vi "Convert Unit (DBL Array).vi"(4 "Quantity":T1, 5 "error in (no error)":errorcluster, 6 "Target Unit":T2, 7 "Base Unit":T2, 8 "Data":dbl[](array[numeric])) -> (0 "error out":errorcluster, 3 "Converted Data":dbl[](array[numeric]))   [LabVIEW 2023, in "NI_HFNetworkAnalysis.lvlib"]
doc: "Convert an array of double values for a specified quantity from a base unit to a new unit."
uses:
  NI_HFNetworkAnalysis.lvlib
  Controls/Unit.ctl
  Controls/Quantity.ctl
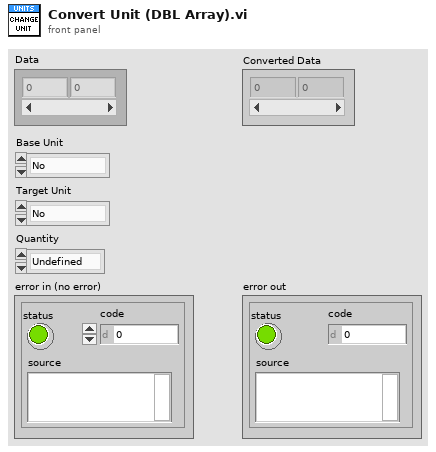
[diagram p1: front panel]
types:
  T1 = typedef "NI_HFNetworkAnalysis.lvlib/Quantity.ctl" = enum16{"Undefined", "V", "I", "A", "B", "P", "Z", "PowerRatio", "Gamma", "Index"}
  T2 = typedef "NI_HFNetworkAnalysis.lvlib/Unit.ctl" = enum16{"No", "s", "Hz", "V", "A", "Ohm", "W", "dB", "dBV", "dBA", "dBm", "percent", "rad", "deg"}
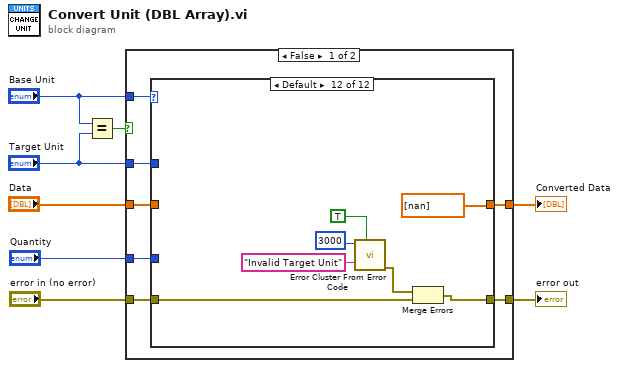
[diagram p0: block diagram]
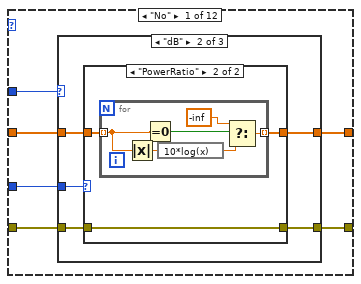
[diagram p2: hidden frame]
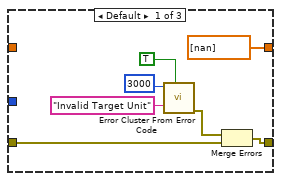
[diagram p3: hidden frame]
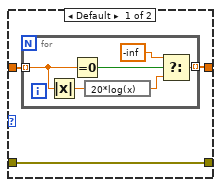
[diagram p4: hidden frame]
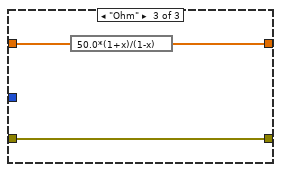
[diagram p5: hidden frame]
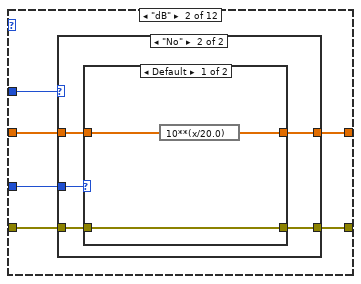
[diagram p6: hidden frame]
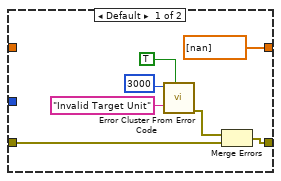
[diagram p7: hidden frame]
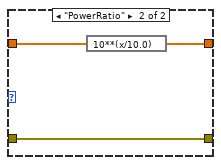
[diagram p8: hidden frame]
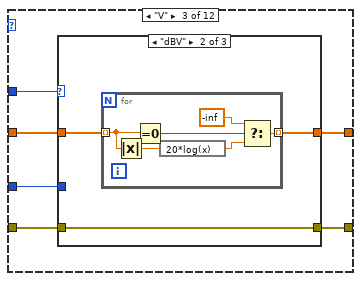
[diagram p9: hidden frame]
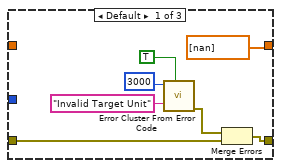
[diagram p10: hidden frame]
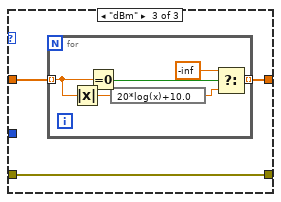
[diagram p11: hidden frame]
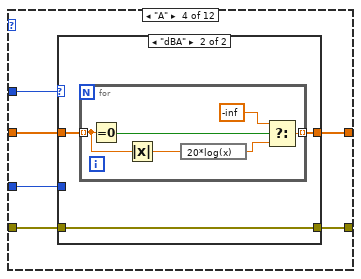
[diagram p12: hidden frame]
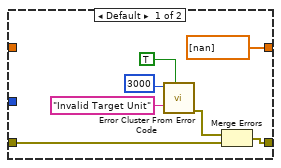
[diagram p13: hidden frame]
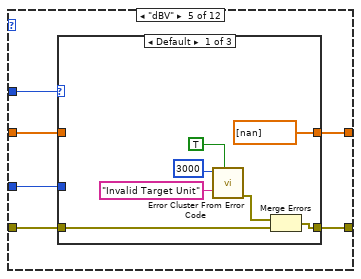
[diagram p14: hidden frame]
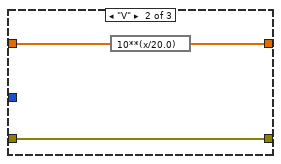
[diagram p15: hidden frame]
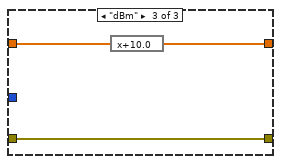
[diagram p16: hidden frame]
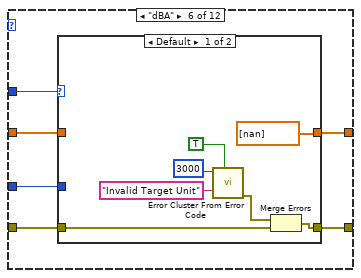
[diagram p17: hidden frame]
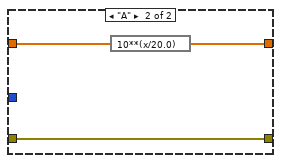
[diagram p18: hidden frame]
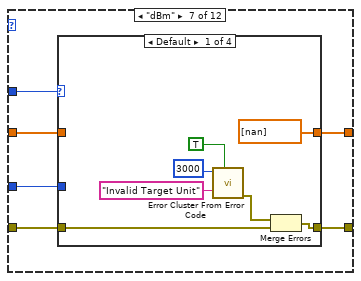
[diagram p19: hidden frame]
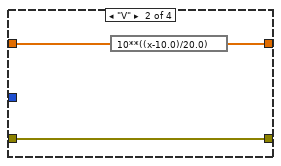
[diagram p20: hidden frame]
diagram:
  n1 = Equal?(x="Base Unit", y="Target Unit") -> (x = y?=w8:bool)
  n2 = case shown="False" w8 {
    tunnel: "Base Unit" -> [w15 _]
    tunnel: [w10 w267] -> w5
    tunnel: "Data" -> [w11 w267]
    tunnel: "Quantity" -> [w14 _]
    tunnel: "error in (no error)" -> [w13 w266]
    tunnel: [w12 w266] -> w2
    tunnel: "Target Unit" -> [w9 _]
    frame False {
      n3 = case shown="Default" w15 {
        tunnel: w14 -> [w21 w60 w84 w115 w137 w156 w172 w194 w215 w231 w247 _]
        tunnel: w13 -> [w20 w59 w83 w114 w136 w155 w171 w193 w214 w230 w246 w265]
        tunnel: [w19 w58 w82 w113 w135 w154 w170 w192 w213 w229 w245 w264] -> w12
        tunnel: w11 -> [w18 w57 w81 w112 w134 w153 w169 w191 w212 w228 w244 _]
        tunnel: [w17 w56 w80 w111 w133 w152 w168 w190 w211 w227 w243 dbl[] [nan] ("Data")] -> w10
        tunnel: w9 -> [w16 w55 w79 w110 w132 w151 w167 w189 w210 w226 w242 _]
        frame "No" {
          n4 = case shown="\"dB\"" w16 {
            tunnel: w21 -> [_ w33 _]
            tunnel: w20 -> [w27 w32 w52]
            tunnel: [w28 w31 w52] -> w19
            tunnel: w18 -> [_ w30 w54]
            tunnel: [dbl[] [nan] ("Data") w29 w53] -> w17
            frame Default {
              n5 = call <vilib>:"Error Cluster From Error Code.vi"("show call chain? (False)"=TRUE, "error message (\"\")"="Invalid Target Unit" ("error message (\"\")"), "error code (0)"=3000) -> ("error out"=w26:errorcluster)  [unwired: 6 in]
              n6 = Merge Errors(w26, w27) -> (w28:errorcluster)
            }
            frame "dB" {
              n7 = case shown="\"PowerRatio\"" w33 {
                tunnel: [w36 w45] -> w31
                tunnel: w32 -> [w36 w45]
                tunnel: w30 -> [w34 w44]
                tunnel: [w35 w43] -> w29
                frame Default {
                  n8 = for {
                    tunnel: [w41] -> w35 mode=indexing
                    tunnel: w34 -> [w38] mode=indexing
                    n9 = Absolute Value(x=w38) -> (abs(x)=w42:dbl)
                    n10 = Equal To 0?(x=w38) -> (x = 0?=w39:bool)
                    n11 = expression code="20*log(x)"(w42) -> (w40:dbl)
                    n12 = Select(t=-inf, s=w39, f=w40) -> (s? t:f=w41:dbl)
                  }
                }
                frame "PowerRatio" {
                  n13 = for {
                    tunnel: w44 -> [w50] mode=indexing
                    tunnel: [w49] -> w43 mode=indexing
                    n14 = Absolute Value(x=w50) -> (abs(x)=w51:dbl)
                    n15 = Equal To 0?(x=w50) -> (x = 0?=w47:bool)
                    n16 = expression code="10*log(x)"(w51) -> (w48:dbl)
                    n17 = Select(t=-inf, s=w47, f=w48) -> (s? t:f=w49:dbl)
                  }
                }
              }
            }
            frame "Ohm" {
              n18 = expression code="50.0*(1+x)/(1-x)"(w54) -> (w53:dbl[])
            }
          }
        }
        frame "dB" {
          n19 = case shown="\"No\"" w55 {
            tunnel: w60 -> [_ w72]
            tunnel: w59 -> [w66 w71]
            tunnel: [w67 w70] -> w58
            tunnel: w57 -> [_ w69]
            tunnel: [dbl[] [nan] ("Data") w68] -> w56
            frame Default {
              n20 = call <vilib>:"Error Cluster From Error Code.vi"("show call chain? (False)"=TRUE, "error message (\"\")"="Invalid Target Unit" ("error message (\"\")"), "error code (0)"=3000) -> ("error out"=w65:errorcluster)  [unwired: 6 in]
              n21 = Merge Errors(w65, w66) -> (w67:errorcluster)
            }
            frame "No" {
              n22 = case shown="Default" w72 {
                tunnel: [w75 w78] -> w70
                tunnel: w71 -> [w75 w78]
                tunnel: w69 -> [w74 w77]
                tunnel: [w73 w76] -> w68
                frame Default {
                  n23 = expression code="10**(x/20.0)"(w74) -> (w73:dbl[])
                }
                frame "PowerRatio" {
                  n24 = expression code="10**(x/10.0)"(w77) -> (w76:dbl[])
                }
              }
            }
          }
        }
        frame "V" {
          n25 = case shown="\"dBV\"" w79 {
            tunnel: w84 -> [_ _ _]
            tunnel: w83 -> [w90 w94 w103]
            tunnel: [w91 w94 w103] -> w82
            tunnel: w81 -> [_ w93 w102]
            tunnel: [dbl[] [nan] ("Data") w92 w101] -> w80
            frame Default {
              n26 = call <vilib>:"Error Cluster From Error Code.vi"("show call chain? (False)"=TRUE, "error message (\"\")"="Invalid Target Unit" ("error message (\"\")"), "error code (0)"=3000) -> ("error out"=w89:errorcluster)  [unwired: 6 in]
              n27 = Merge Errors(w89, w90) -> (w91:errorcluster)
            }
            frame "dBV" {
              n28 = for {
                tunnel: w93 -> [w99] mode=indexing
                tunnel: [w95] -> w92 mode=indexing
                n29 = Absolute Value(x=w99) -> (abs(x)=w100:dbl)
                n30 = Equal To 0?(x=w99) -> (x = 0?=w97:bool)
                n31 = expression code="20*log(x)"(w100) -> (w98:dbl)
                n32 = Select(t=-inf, s=w97, f=w98) -> (s? t:f=w95:dbl)
              }
            }
            frame "dBm" {
              n33 = for {
                tunnel: w102 -> [w108] mode=indexing
                tunnel: [w106] -> w101 mode=indexing
                n34 = Absolute Value(x=w108) -> (abs(x)=w109:dbl)
                n35 = Equal To 0?(x=w108) -> (x = 0?=w105:bool)
                n36 = expression code="20*log(x)+10.0"(w109) -> (w107:dbl)
                n37 = Select(t=-inf, s=w105, f=w107) -> (s? t:f=w106:dbl)
              }
            }
          }
        }
        frame "A" {
          n38 = case shown="\"dBA\"" w110 {
            tunnel: w115 -> [_ _]
            tunnel: w114 -> [w121 w125]
            tunnel: [w122 w125] -> w113
            tunnel: w112 -> [_ w124]
            tunnel: [dbl[] [nan] ("Data") w123] -> w111
            frame Default {
              n39 = call <vilib>:"Error Cluster From Error Code.vi"("show call chain? (False)"=TRUE, "error message (\"\")"="Invalid Target Unit" ("error message (\"\")"), "error code (0)"=3000) -> ("error out"=w120:errorcluster)  [unwired: 6 in]
              n40 = Merge Errors(w120, w121) -> (w122:errorcluster)
            }
            frame "dBA" {
              n41 = for {
                tunnel: w124 -> [w130] mode=indexing
                tunnel: [w127] -> w123 mode=indexing
                n42 = Equal To 0?(x=w130) -> (x = 0?=w128:bool)
                n43 = Absolute Value(x=w130) -> (abs(x)=w131:dbl)
                n44 = expression code="20*log(x)"(w131) -> (w129:dbl)
                n45 = Select(t=-inf, s=w128, f=w129) -> (s? t:f=w127:dbl)
              }
            }
          }
        }
        frame "dBV" {
          n46 = case shown="Default" w132 {
            tunnel: w137 -> [_ _ _]
            tunnel: w136 -> [w143 w147 w150]
            tunnel: [w144 w147 w150] -> w135
            tunnel: w134 -> [_ w146 w149]
            tunnel: [dbl[] [nan] ("Data") w145 w148] -> w133
            frame Default {
              n47 = call <vilib>:"Error Cluster From Error Code.vi"("show call chain? (False)"=TRUE, "error message (\"\")"="Invalid Target Unit" ("error message (\"\")"), "error code (0)"=3000) -> ("error out"=w142:errorcluster)  [unwired: 6 in]
              n48 = Merge Errors(w142, w143) -> (w144:errorcluster)
            }
            frame "V" {
              n49 = expression code="10**(x/20.0)"(w146) -> (w145:dbl[])
            }
            frame "dBm" {
              n50 = expression code="x+10.0"(w149) -> (w148:dbl[])
            }
          }
        }
        frame "dBA" {
          n51 = case shown="Default" w151 {
            tunnel: w156 -> [_ _]
            tunnel: w155 -> [w162 w166]
            tunnel: [w163 w166] -> w154
            tunnel: w153 -> [_ w165]
            tunnel: [dbl[] [nan] ("Data") w164] -> w152
            frame Default {
              n52 = call <vilib>:"Error Cluster From Error Code.vi"("show call chain? (False)"=TRUE, "error message (\"\")"="Invalid Target Unit" ("error message (\"\")"), "error code (0)"=3000) -> ("error out"=w161:errorcluster)  [unwired: 6 in]
              n53 = Merge Errors(w161, w162) -> (w163:errorcluster)
            }
            frame "A" {
              n54 = expression code="10**(x/20.0)"(w165) -> (w164:dbl[])
            }
          }
        }
        frame "dBm" {
          n55 = case shown="Default" w167 {
            tunnel: w172 -> [_ _ _ _]
            tunnel: w171 -> [w178 w182 w185 w188]
            tunnel: [w179 w182 w185 w188] -> w170
            tunnel: w169 -> [_ w181 w184 w187]
            tunnel: [dbl[] [nan] ("Data") w180 w183 w186] -> w168
            frame Default {
              n56 = call <vilib>:"Error Cluster From Error Code.vi"("show call chain? (False)"=TRUE, "error message (\"\")"="Invalid Target Unit" ("error message (\"\")"), "error code (0)"=3000) -> ("error out"=w177:errorcluster)  [unwired: 6 in]
              n57 = Merge Errors(w177, w178) -> (w179:errorcluster)
            }
            frame "V" {
              n58 = expression code="10**((x-10.0)/20.0)"(w181) -> (w180:dbl[])
            }
            frame "dBV" {
              n59 = expression code="x-10.0"(w184) -> (w183:dbl[])
            }
            frame "W" {
              n60 = expression code="10**((x-30.0)/10.0)"(w187) -> (w186:dbl[])
            }
          }
        }
        frame "W" {
          n61 = case shown="\"dBm\"" w189 {
            tunnel: w194 -> [_ _]
            tunnel: w193 -> [w200 w204]
            tunnel: [w201 w204] -> w192
            tunnel: w191 -> [_ w203]
            tunnel: [dbl[] [nan] ("Data") w202] -> w190
            frame Default {
              n62 = call <vilib>:"Error Cluster From Error Code.vi"("show call chain? (False)"=TRUE, "error message (\"\")"="Invalid Target Unit" ("error message (\"\")"), "error code (0)"=3000) -> ("error out"=w199:errorcluster)  [unwired: 6 in]
              n63 = Merge Errors(w199, w200) -> (w201:errorcluster)
            }
            frame "dBm" {
              n64 = for {
                tunnel: w203 -> [w209] mode=indexing
                tunnel: [w205] -> w202 mode=indexing
                n65 = Equal To 0?(x=w209) -> (x = 0?=w207:bool)
                n66 = expression code="30.0+10*log(x)"(w209) -> (w208:dbl)
                n67 = Select(t=-inf, s=w207, f=w208) -> (s? t:f=w205:dbl)
              }
            }
          }
        }
        frame "rad" {
          n68 = case shown="\"deg\"" w210 {
            tunnel: w215 -> [_ _]
            tunnel: w214 -> [w221 w225]
            tunnel: [w222 w225] -> w213
            tunnel: w212 -> [_ w224]
            tunnel: [dbl[] [nan] ("Data") w223] -> w211
            frame Default {
              n69 = call <vilib>:"Error Cluster From Error Code.vi"("show call chain? (False)"=TRUE, "error message (\"\")"="Invalid Target Unit" ("error message (\"\")"), "error code (0)"=3000) -> ("error out"=w220:errorcluster)  [unwired: 6 in]
              n70 = Merge Errors(w220, w221) -> (w222:errorcluster)
            }
            frame "deg" {
              n71 = expression code="(x/pi)*180.0" ("radians to degrees")(w224) -> (w223:dbl[])
            }
          }
        }
        frame "deg" {
          n72 = case shown="\"rad\"" w226 {
            tunnel: w231 -> [_ _]
            tunnel: w230 -> [w237 w241]
            tunnel: [w238 w241] -> w229
            tunnel: w228 -> [_ w240]
            tunnel: [dbl[] [nan] ("Data") w239] -> w227
            frame Default {
              n73 = call <vilib>:"Error Cluster From Error Code.vi"("show call chain? (False)"=TRUE, "error message (\"\")"="Invalid Target Unit" ("error message (\"\")"), "error code (0)"=3000) -> ("error out"=w236:errorcluster)  [unwired: 6 in]
              n74 = Merge Errors(w236, w237) -> (w238:errorcluster)
            }
            frame "rad" {
              n75 = expression code="(x/180.0)*pi" ("radians to degrees")(w240) -> (w239:dbl[])
            }
          }
        }
        frame "Ohm" {
          n76 = case shown="\"No\"" w242 {
            tunnel: w247 -> [_ _]
            tunnel: w246 -> [w253 w258]
            tunnel: [w254 w258] -> w245
            tunnel: w244 -> [_ w256]
            tunnel: [dbl[] [nan] ("Data") w257] -> w243
            frame Default {
              n77 = call <vilib>:"Error Cluster From Error Code.vi"("show call chain? (False)"=TRUE, "error message (\"\")"="Invalid Target Unit" ("error message (\"\")"), "error code (0)"=3000) -> ("error out"=w252:errorcluster)  [unwired: 6 in]
              n78 = Merge Errors(w252, w253) -> (w254:errorcluster)
            }
            frame "No" {
              n79 = expression code="x/50.0"(w256) -> (w255:dbl[])
              n80 = expression code="(x-1)/(x+1)"(w255) -> (w257:dbl[])
            }
          }
        }
        frame Default {
          n81 = call <vilib>:"Error Cluster From Error Code.vi"("show call chain? (False)"=TRUE, "error message (\"\")"="Invalid Target Unit" ("error message (\"\")"), "error code (0)"=3000) -> ("error out"=w263:errorcluster)  [unwired: 6 in]
          n82 = Merge Errors(w263, w265) -> (w264:errorcluster)
        }
      }
    }
    frame True {
    }
  }
  "Converted Data" <- w5
  "error out" <- w2
